vi "applyDistanceGaugePreset.vi"(8 "error in (no error)":errorcluster, 11 "Model in":refnum<class "Model.lvclass">) -> (0 "error out":errorcluster, 3 "Model out":refnum<class "Model.lvclass">)   [LabVIEW 2015, in "Model.lvclass"]
uses:
  Model.lvclass
  Model.lvclass/Model.ctl
  <userlib>/Common/Devices/DistanceGauge/DistanceGauge/DistanceGauge.lvclass
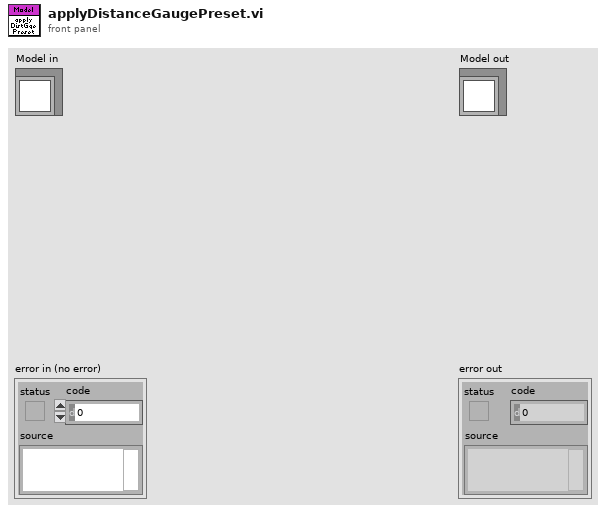
[diagram p1: front panel]
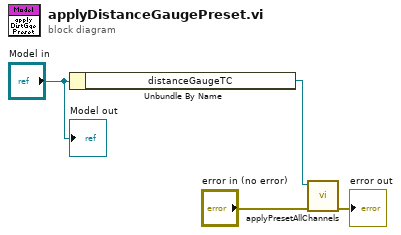
[diagram p0: block diagram]
diagram:
  n1 = Unbundle By Name("Model in") -> ("distanceGaugeTC"=w4:refnum<class "DistanceGaugeTC.lvclass">)
  n2 = call <userlib>:"applyPresetAllChannels.vi"("error in (no error)"="error in (no error)", "DistanceGauge in"=w4) -> ("error out"=→"error out":errorcluster)  [unwired: 8 in, 1 out]
  "Model out" <- "Model in"
